vi "CumulativePowerSpectrum.vi"(8 "error in (no error)":errorcluster, 11 "PSD":cluster{"f0":dbl, "df":dbl, "magnitude":dbl[]} {"f0" format="%0.2p"; "df" format="%0.2p"; "magnitude" format="%.2p"}) -> (0 "error out":errorcluster, 3 "CPS":cluster{"f0":dbl, "df":dbl, "magnitude":dbl[]} {"f0" format="%0.2p"; "df" format="%0.2p"; "magnitude" format="%.2p"})   [LabVIEW 2018, in "Spectra.lvlib"]
doc: "CPS takes the power spectral density data and returns the Cumulative Power Spectrum of the signal.\n\nThe start and end points are adjusted to match the dc power and the total power respectively."
uses:
  Spectra.lvlib
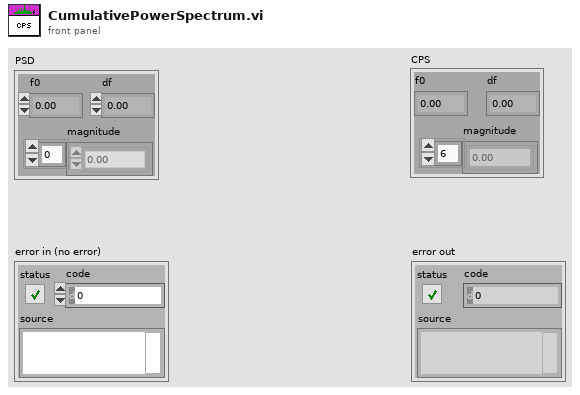
[diagram p1: front panel]
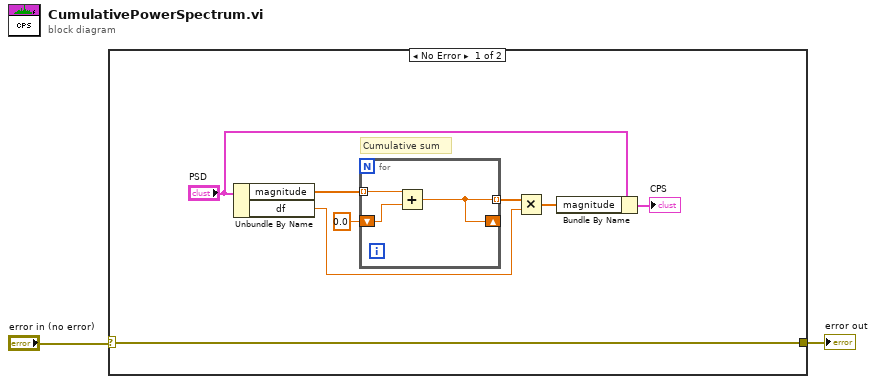
[diagram p0: block diagram]
diagram:
  n1 = case shown="No Error" "error in (no error)" {
    selector: "error in (no error)" -> [w3 w14]
    tunnel: [w3 w14] -> w1
    frame No Error {
      # "Cumulative sum"
      n2 = Unbundle By Name("PSD") -> ("magnitude"=w8:dbl[], "df"=w6:dbl)
      n3 = for {
        tunnel: [w13] -> w5 mode=indexing
        shift-right: [w13] -> _
        shift-left: 0.0 -> [w12]
        tunnel: w8 -> [w11] mode=indexing
        n4 = Add(x=w11, y=w12) -> (x+y=w13:dbl)
      }
      n5 = Multiply(x=w5, y=w6) -> (x*y=w4:dbl[])
      n6 = Bundle By Name(cluster="PSD", "magnitude"=w4) -> (→"CPS":cluster{"f0":dbl, "df":dbl, "magnitude":dbl[]})
    }
    frame Error {
    }
  }
  "error out" <- w1
